vi "To Pretty String.vi"(8 "error in (no error)":errorcluster, 11 "JSON Boolean in":refnum<class "JSON Boolean.lvclass">) -> (0 "error out":errorcluster, 3 "Pretty Print String":string)   [LabVIEW 2017]
uses:
  JSON Boolean.lvclass
  LVJSON.lvlib
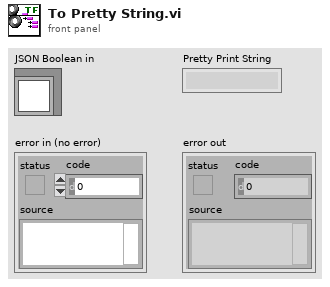
[diagram p1: front panel]
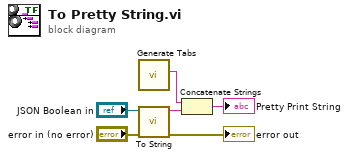
[diagram p0: block diagram]
diagram:
  n1 = call "Generate Tabs.vi"() -> ("Tabs"=w3:string)  [unwired: 10 in, 1 out]
  n2 = call-dynamic "To String.vi"("error in (no error)"="error in (no error)", "JSON Boolean in"="JSON Boolean in") -> ("error out"=→"error out":errorcluster, "String"=w2:string)  [unwired: 8 in]
  n3 = Concatenate Strings(w3, w2) -> (→"Pretty Print String":string)
